vi "ImPro - Settings Manager.vi"(7 "Command":enum16{"Read", "Write"}(ring), 8 "error in (no error)":errorcluster, 10 "ImagePath":path, 11 "ImProSettings In":T1) -> (0 "error out":errorcluster, 3 "ImProSettings Out":T1)   [LabVIEW 2023]
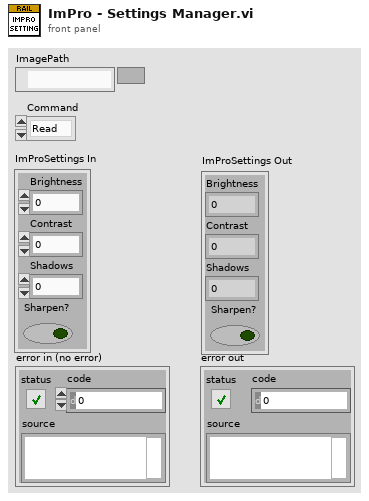
[diagram p1: front panel]
types:
  T1 = cluster{"Brightness":dbl, "Contrast":dbl, "Shadows":dbl, "Sharpen?":bool}
  T2 = enum16{"open", "replace", "create", "open or create", "replace or create", "replace or create with confirmation"}
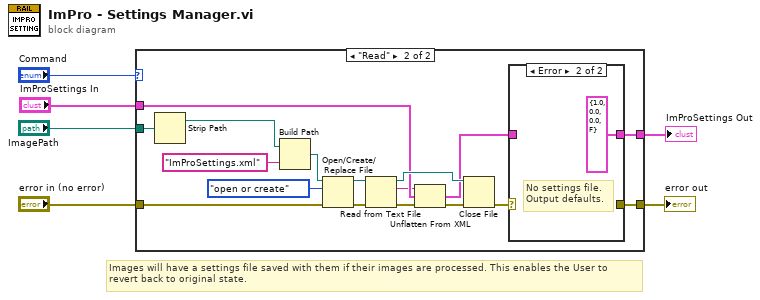
[diagram p0: block diagram]
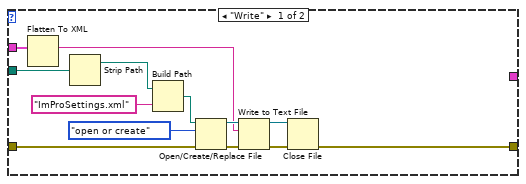
[diagram p2: hidden frame]
diagram:
  # "Images will have a settings file saved with them if their images are processed. This enables the User to\nrevert back to original state."
  n1 = case shown="\"Read\"" "Command" {
    tunnel: "ImagePath" -> [w19 w36]
    tunnel: "error in (no error)" -> [w16 w33]
    tunnel: "ImProSettings In" -> [w9 w25]
    tunnel: [w7 w20] -> w6
    tunnel: [_ w22] -> w1
    frame "Write" {
      n2 = Flatten To XML(6:w9) -> (2:w8:string)
      n3 = Strip Path(path=w19) -> (stripped path=w18:path)  [unwired: 1 out]
      n4 = Build Path(base path=w18, name or relative path="ImProSettings.xml") -> (appended path=w15:path)
      n5 = Open/Create/Replace File(file path (use dialog)=w15, error in=w16, operation (0:open)=T2."open or create") -> (refnum out=w12:refnum<file>, error out=w13:errorcluster)  [unwired: 3 in, 1 out]
      n6 = Write to Text File(file (use dialog)=w12, text=w8, error in=w13) -> (refnum out=w10:refnum<file>, error out=w11:errorcluster)  [unwired: 1 in, 1 out]
      n7 = Close File(refnum=w10, error in=w11) -> (error out=w7:errorcluster)  [unwired: 1 out]
    }
    frame "Read" {
      n8 = Strip Path(path=w36) -> (stripped path=w35:path)  [unwired: 1 out]
      n9 = Build Path(base path=w35, name or relative path="ImProSettings.xml") -> (appended path=w32:path)
      n10 = Open/Create/Replace File(file path (use dialog)=w32, error in=w33, operation (0:open)=T2."open or create") -> (refnum out=w29:refnum<file>, error out=w30:errorcluster)  [unwired: 3 in, 1 out]
      n11 = Read from Text File(file (use dialog)=w29, error in=w30) -> (refnum out=w28:refnum<file>, text=w24:string, error out=w27:errorcluster)  [unwired: 2 in, 1 out]
      n12 = Unflatten From XML(xml string=w24, type=w25, error in (no error)=w27) -> (value=w21:T1, error out=w26:errorcluster)
      n13 = Close File(refnum=w28, error in=w26) -> (error out=w23:errorcluster)  [unwired: 1 out]
      n14 = case shown="Error" w23 {
        selector: w23 -> [w37 _]
        tunnel: [w38 T1 {"Brightness"=1.0, "Contrast"=0.0, "Shadows"=0.0, "Sharpen?"=FALSE} ("ImProSettings In")] -> w22
        tunnel: w21 -> [w38 _]
        tunnel: [w37 _] -> w20
        frame No Error {
        }
        frame Error {
          # "No settings file.\nOutput defaults."
        }
      }
    }
  }
  "error out" <- w6
  "ImProSettings Out" <- w1
